vi "Read ext_stop.vi"(8 "error in (no error)":errorcluster, 11 "Calibration Actor in":refnum<class "Calibration Actor.lvclass">) -> (0 "error out":errorcluster, 2 "ext_stop":refnum<k4>, 3 "Calibration Actor out":refnum<class "Calibration Actor.lvclass">)   [LabVIEW 2014, in "Calibration.lvlib" / "Calibration Actor.lvclass"]
uses:
  Calibration Actor.lvclass
  Calibration Actor.lvclass/Calibration Actor.ctl
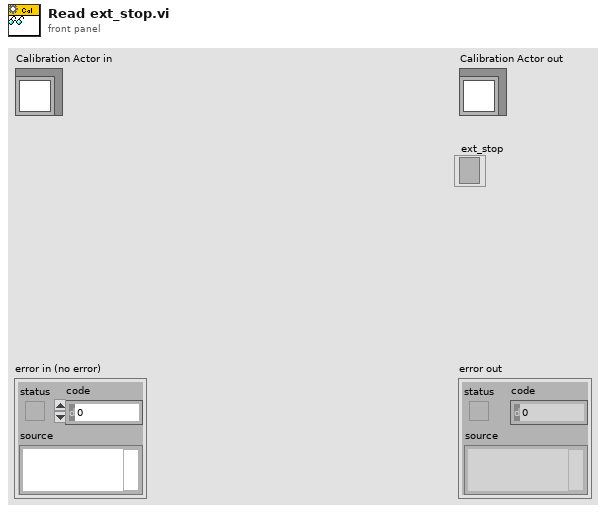
[diagram p1: front panel]
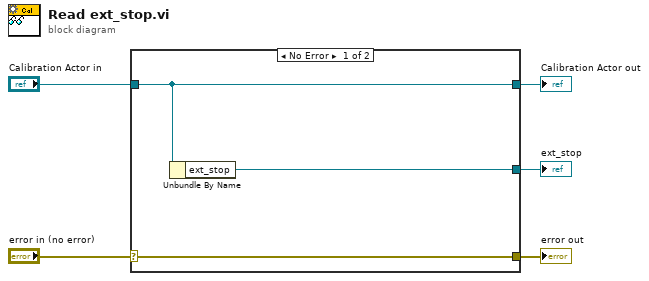
[diagram p0: block diagram]
diagram:
  n1 = case shown="No Error" "error in (no error)" {
    selector: "error in (no error)" -> [w8 w9]
    tunnel: [w8 w9] -> w4
    tunnel: [w7 w10] -> w2
    tunnel: "Calibration Actor in" -> [w7 w10]
    tunnel: [w6 _] -> w1
    frame No Error {
      n2 = Unbundle By Name(w7) -> ("ext_stop"=w6:refnum<k4>)
    }
    frame Error {
    }
  }
  "error out" <- w4
  "Calibration Actor out" <- w2
  "ext_stop" <- w1
